vi "Export Instrument Addon Configuration.vi"(8 "Error In":errorcluster, 10 "Exported File Path":path, 11 "Instrument Addon Refnum In":T1=18446744073709551615 format="%.0x") -> (0 "Error Out":errorcluster, 3 "Instrument Addon Refnum Out":T1=18446744073709551615 format="%.0x")   [LabVIEW 2020, in "Scripting API.lvlib"]
uses:
  Scripting API.lvlib
  <vilib>/NI VeriStand/Custom Device API/Custom Device Item Ref.ctl
  <vilib>/NI VeriStand/Custom Device API/Custom Device API.lvlib
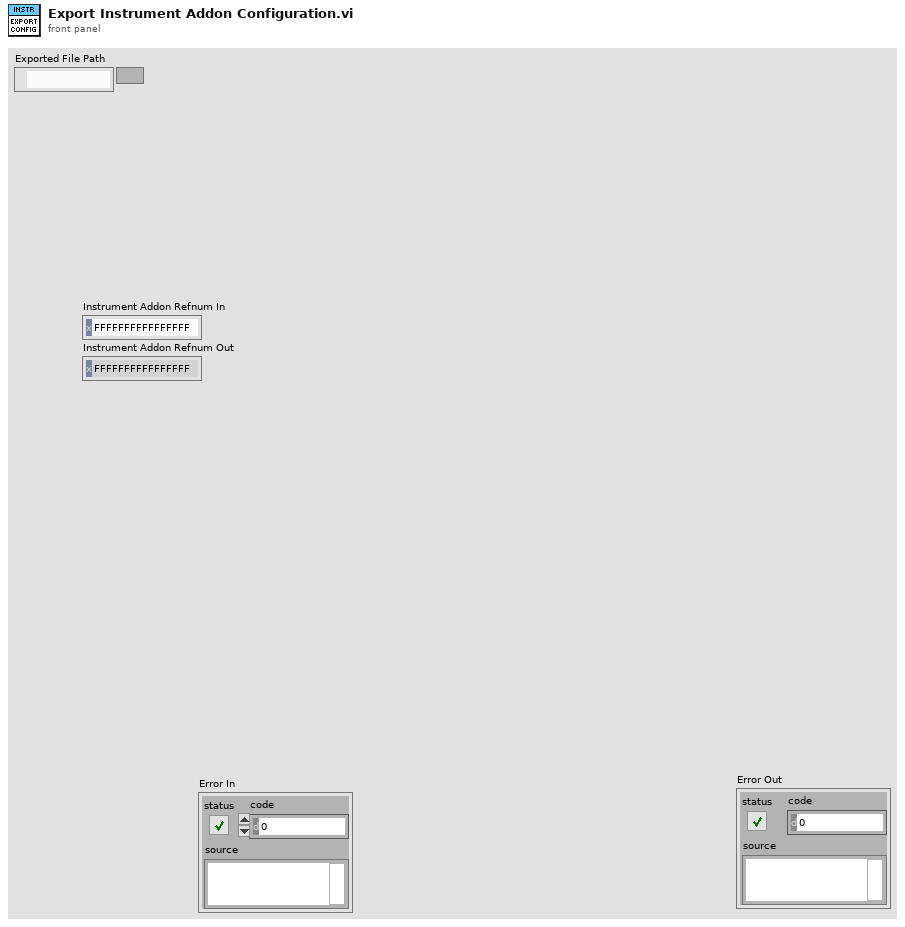
[diagram p1: front panel]
types:
  T1 = typedef "Custom Device API.lvlib/Custom Device Item Ref.ctl" = u64
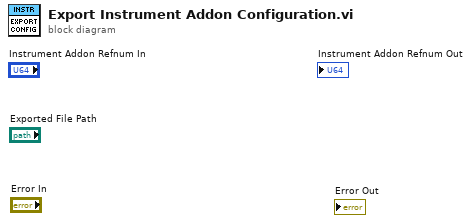
[diagram p0: block diagram]
diagram:
